vi "HRTF-Plot Response.vi"(0 "Cal.Data in":T2, 2 "State":T1, 11 "error in (no error)":errorcluster) -> (4 "Cal.Data out":T2, 6 "time":cluster{"offset":dbl, "dx":dbl, "Y":dbl[][]}, 8 "crosscorr":cluster{"offset":dbl, "dx":dbl, "Y":dbl[][]}, 13 "phase":cluster{"offset":dbl, "dx":dbl, "Y":dbl[][]}, 14 "mag":cluster{"offset":dbl, "dx":dbl, "Y":dbl[][]}, 15 "error out":errorcluster)   [LabVIEW 2015]
uses:
  Typedefs/HRTF-Runtime Data.ctl
  Typedefs/HRTF-State.ctl
  <vilib>/Analysis/2dsp.llb/Complex FFT.vi
  <vilib>/Analysis/2dsp.llb/Inverse Real FFT.vi
  PXI DAQ VIs/Utility VIs/Array Dimensions (2D).vi
  Utility VIs/Math VIs/FFT x(t) to dB,Degrees (2D).vi
  Utility VIs/Conversion VIs/Create Waveform Cluster (2D).vi
  <vilib>/Analysis/NI_AALPro.lvlib
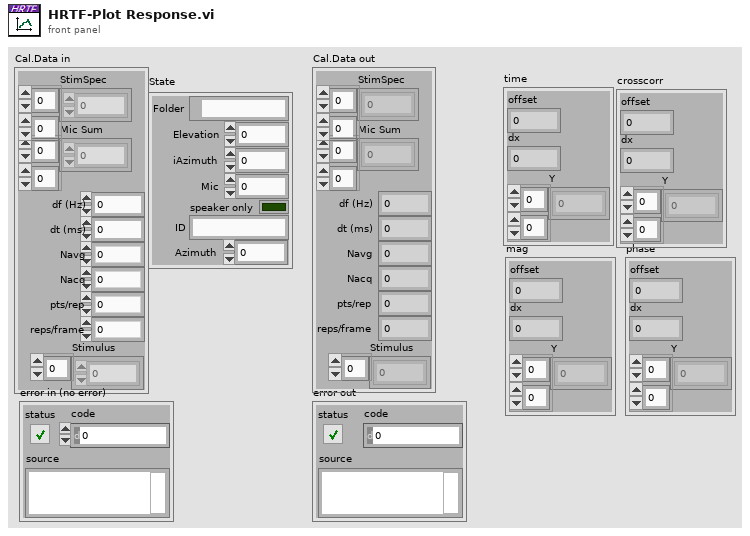
[diagram p1: front panel]
types:
  T1 = typedef "HRTF-State.ctl" = cluster{"Folder":path, "Elevation":dbl, "iAzimuth":i32, "Mic":i32, "speaker only":bool, "ID":string, "Azimuth":dbl}
  T2 = typedef "HRTF-Runtime Data.ctl" = cluster{"StimSpec":cdb[][], "Mic Sum":dbl[][], "df (Hz)":dbl, "dt (ms)":dbl, "Navg":i32, "Nacq":i32, "pts/rep":i32, "reps/frame":i32, "Stimulus":dbl[]}
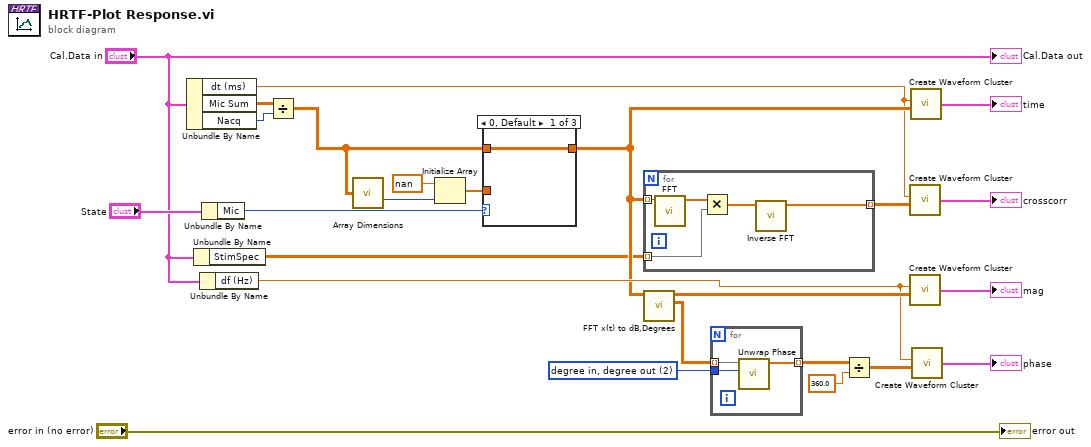
[diagram p0: block diagram]
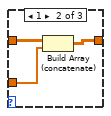
[diagram p2: hidden frame]
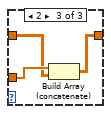
[diagram p3: hidden frame]
diagram:
  w17 = 2 items=["radian in, radian out", "radian in, degree out", "degree in, degree out", "degree in, radian out"] ("phase unit")
  n1 = Unbundle By Name("Cal.Data in") -> ("dt (ms)"=w7:dbl, "Mic Sum"=w19:dbl[][], "Nacq"=w18:i32)
  n2 = Unbundle By Name("Cal.Data in") -> ("StimSpec"=w6:cdb[][])
  n3 = Unbundle By Name("Cal.Data in") -> ("df (Hz)"=w10:dbl)
  n4 = Unbundle By Name("State") -> ("Mic"=w14:i32)
  n5 = Divide(x=w19, y=w18) -> (x/y=w15:dbl[][])
  n6 = call-poly "Array Dimensions.vi"("2D Array"=w15) -> ("# columns"=w3:i32)  [unwired: 13 in, 1 out]
  n7 = Initialize Array(nan, w3) -> (w1:dbl[])
  n8 = case shown="0, Default" w14 {
    tunnel: w15 -> [w26 w29 w31]
    tunnel: w1 -> [_ w28 w32]
    tunnel: [w26 w27 w30] -> w9
    frame 0, Default {
    }
    frame 1 {
      n9 = Build Array (concatenate)(w29, w28) -> (w27:dbl[][])
    }
    frame 2 {
      n10 = Build Array (concatenate)(w32, w31) -> (w30:dbl[][])
    }
  }
  n11 = for {
    tunnel: w9 -> [w37] mode=indexing
    tunnel: [w36] -> w8 mode=indexing
    tunnel: w6 -> [w34] mode=indexing
    n12 = call-poly <vilib>:"FFT.vi"("X"=w37) -> ("FFT {X}"=w35:cdb[])  [unwired: 9 in, 1 out]
    n13 = Multiply(x=w35, y=w34) -> (x*y=w33:cdb[])
    n14 = call-poly <vilib>:"Inverse FFT.vi"("FFT {X}"=w33) -> ("X"=w36:dbl[])  [unwired: 9 in, 1 out]
  }
  n15 = call-poly "FFT x(t) to dB,Degrees.vi"("X(t)"=w9) -> ("+Freq Phase of FFT (degrees)"=w4:dbl[][], "+Freq. Mag of FFT (dB rms)"=w13:dbl[][])  [unwired: 9 in]
  n16 = for {
    tunnel: w17 -> [w40]
    tunnel: w4 -> [w39] mode=indexing
    tunnel: [w38] -> w12 mode=indexing
    n17 = call <vilib>:"Unwrap Phase.vi"("phase unit"=w40, "Phase"=w39) -> ("Unwrapped Phase"=w38:dbl[])  [unwired: 8 in, 1 out]
  }
  n18 = Divide(x=w12, y=360.0) -> (x/y=w11:dbl[][])
  n19 = call-poly "Create Waveform Cluster.vi"("dx"=w7, "Array"=w8) -> ("waveform cluster"=→"crosscorr":cluster{"offset":dbl, "dx":dbl, "Y":dbl[][]})  [unwired: 3 in]
  n20 = call-poly "Create Waveform Cluster.vi"("dx"=w10, "Array"=w13) -> ("waveform cluster"=→"mag":cluster{"offset":dbl, "dx":dbl, "Y":dbl[][]})  [unwired: 3 in]
  n21 = call-poly "Create Waveform Cluster.vi"("dx"=w7, "Array"=w9) -> ("waveform cluster"=→"time":cluster{"offset":dbl, "dx":dbl, "Y":dbl[][]})  [unwired: 3 in]
  n22 = call-poly "Create Waveform Cluster.vi"("dx"=w10, "Array"=w11) -> ("waveform cluster"=→"phase":cluster{"offset":dbl, "dx":dbl, "Y":dbl[][]})  [unwired: 3 in]
  "error out" <- "error in (no error)"
  "Cal.Data out" <- "Cal.Data in"
